vi "VariableGroupsEditUI.vi"(11 "VariableManagerRef in":refnum<vi>) -> (3 "VariableManagerRef out":refnum<vi>)   [LabVIEW 2013]
doc: "Create a window for add/edit variable groups of the given VariableManager reference."
uses:
  VariableGroup/VariableGroup.lvclass
  VariableManager/VariableManager.lvclass
  Variable/Variable.lvclass
  API/VariableManagerAPI.lvlib
panel:
  in  "Delete Button":bool
  in  "Rename Button":bool
  in  "Add Button":bool
  in  "InputName":string caption="Input Group Name"
  in  "VariableNames":string[](array[string])
  in  "VariableGroups":refnum<class "VariableGroup.lvclass">[](array[class])
  in  "OK Button":bool
  in  "Cancel Button":bool
  in  "Exclude":bool
  in  "Include":bool
  in  "IncludedVariables":i32[](listbox) caption="Included Variables"
  in  "ExcludedVariables":i32[](listbox) caption="Excluded Variables"
  in  "VariableGroup":u16(ring) caption="Variable Group"
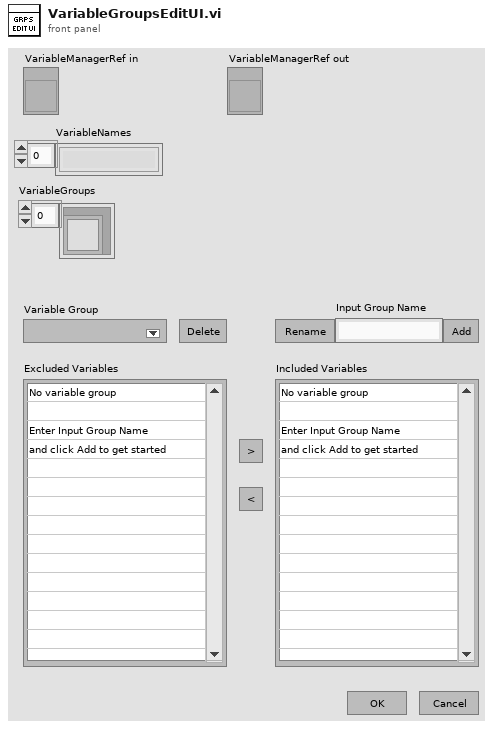
[diagram p1: front panel]
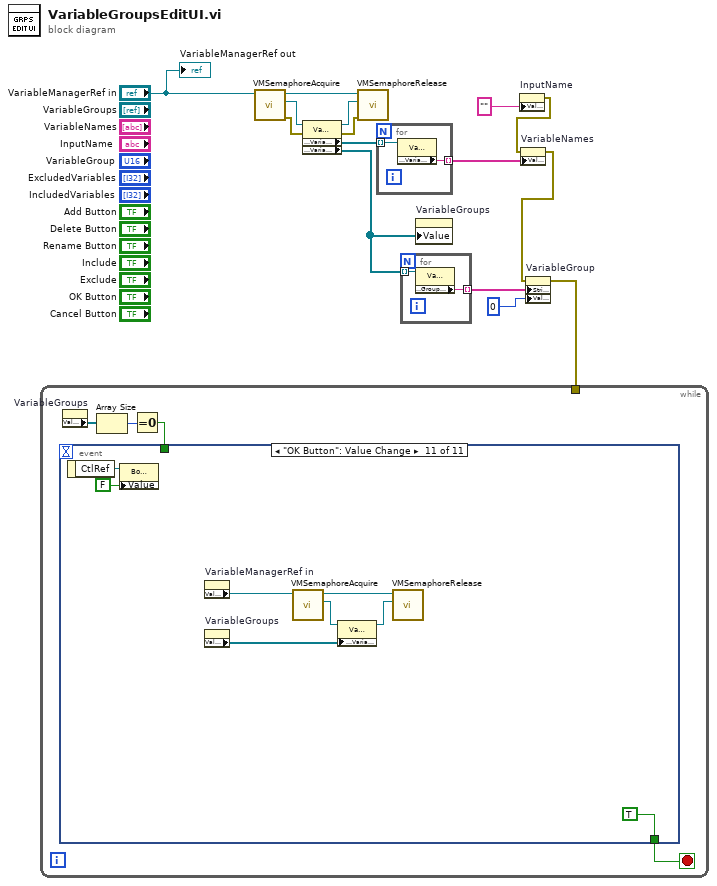
[diagram p0: block diagram]
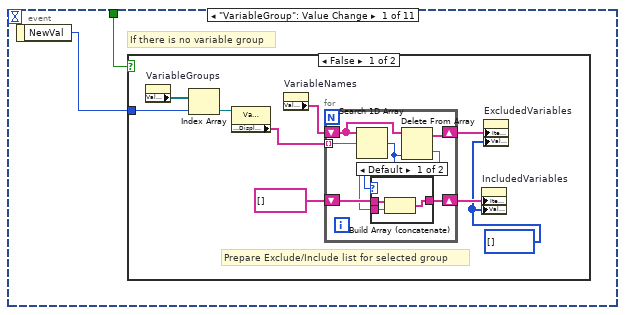
[diagram p2: hidden frame]
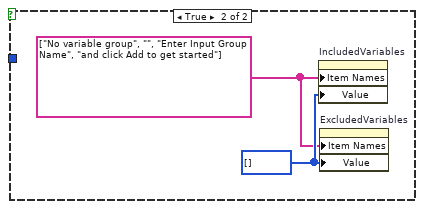
[diagram p4: hidden frame]
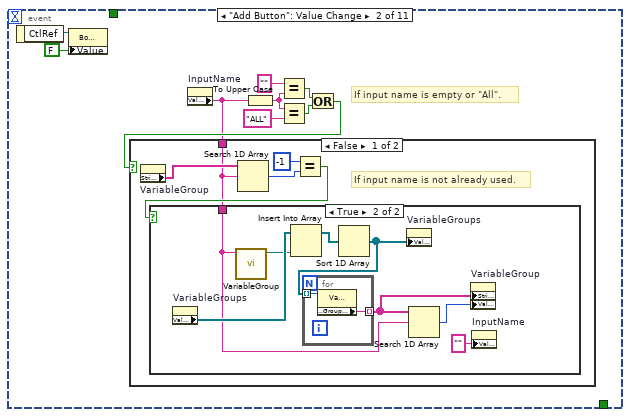
[diagram p5: hidden frame]
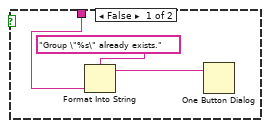
[diagram p6: hidden frame]
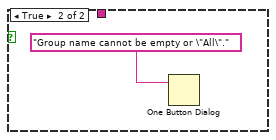
[diagram p7: hidden frame]
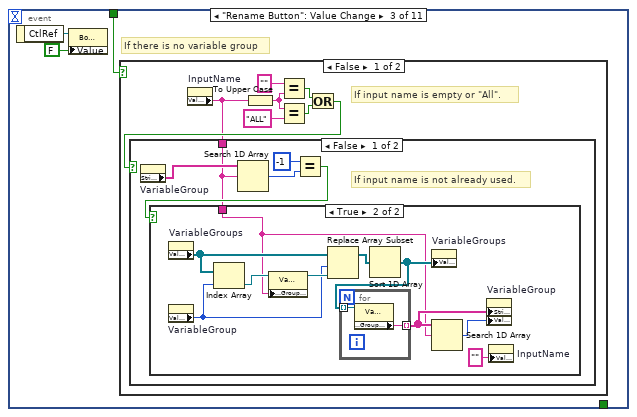
[diagram p8: hidden frame]
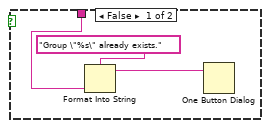
[diagram p9: hidden frame]
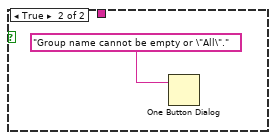
[diagram p10: hidden frame]
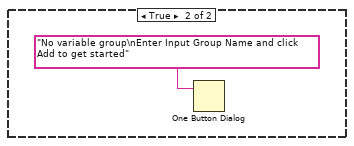
[diagram p11: hidden frame]
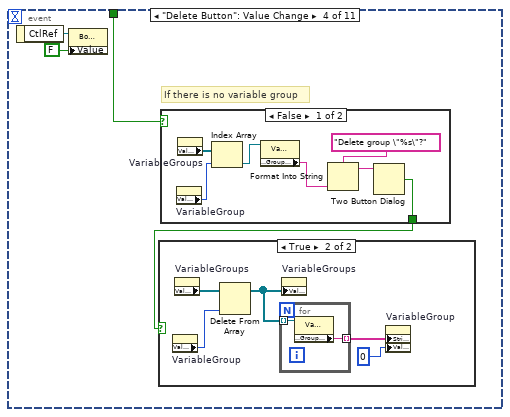
[diagram p12: hidden frame]
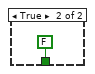
[diagram p13: hidden frame]
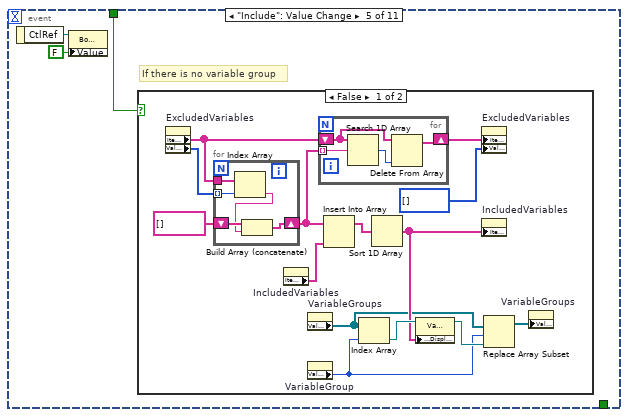
[diagram p15: hidden frame]
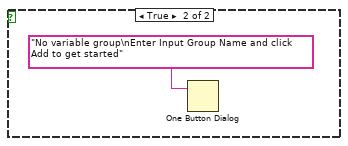
[diagram p16: hidden frame]
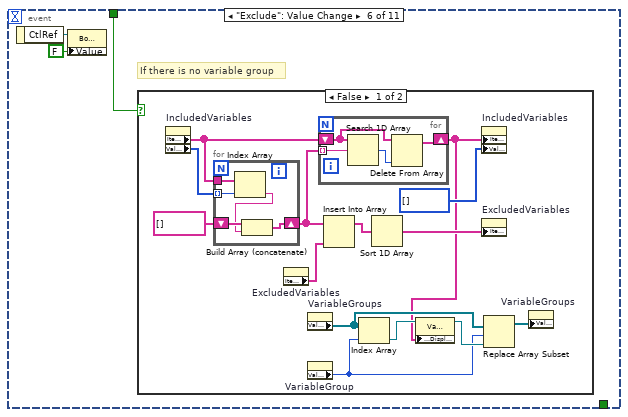
[diagram p17: hidden frame]
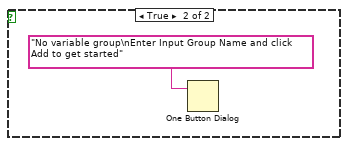
[diagram p18: hidden frame]
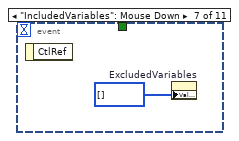
[diagram p19: hidden frame]
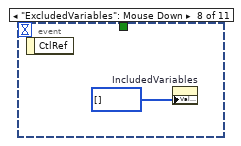
[diagram p20: hidden frame]
diagram:
  n1 = call "VMSemaphoreAcquire.vi"("VariableManagerRef in"="VariableManagerRef in") -> ("error out"=w2:errorcluster, "VariableManager"=w10:refnum<class "VariableManager.lvclass">, "VariableManagerRef out"=w4:refnum<vi>)  [unwired: 7 in, 1 out]
  n2 = property class="VariableManager.lvclass"(reference=w10, error in=w2) -> (reference out=w5:refnum<class "VariableManager.lvclass">, error out=w1:errorcluster, "Accessors:Variables"=w8:refnum<class "Variable.lvclass">[], "Accessors:VariableGroups"=w9:refnum<class "VariableGroup.lvclass">[])
  n3 = call "VMSemaphoreRelease.vi"("error in (no error)"=w1, "VariableManager"=w5, "VariableManagerRef in"=w4) -> ()  [unwired: 7 in, 2 out]
  n4 = for {
    tunnel: w8 -> [w17] mode=indexing
    tunnel: [w16] -> w7 mode=indexing
    n5 = property class="Variable.lvclass"(reference=w17) -> ("Accessors:VariableName"=w16:string)  [unwired: 1 in, 2 out]
  }
  n6 = for {
    tunnel: w9 -> [w19] mode=indexing
    tunnel: [w18] -> w14 mode=indexing
    n7 = property class="VariableGroup.lvclass"(reference=w19) -> ("Accessors:GroupName"=w18:string)  [unwired: 1 in, 2 out]
  }
  n8 = property on="VariableGroups" class="Arr (strict)"("Value"=w9) -> ()  [unwired: 2 in, 2 out]
  n9 = property on="InputName" class="Str"("Value"="") -> (error out=w11:errorcluster)  [unwired: 2 in, 1 out]
  n10 = property on="VariableNames" class="Arr (strict)"(error in=w11, "Value"=w7) -> (error out=w13:errorcluster)  [unwired: 1 in, 1 out]
  n11 = property on="VariableGroup" class="Ring (strict)"(error in=w13, "Strings []"=w14, "Val(Sgnl)"=u16 0 ("Value (Signaling)")) -> (error out=w6:errorcluster)  [unwired: 1 in, 1 out]
  n12 = while {
    tunnel: w6 -> [_]
    stop <- w23 stop-if-true
    n13 = property on="VariableGroups" class="Arr (strict)"() -> ("Value"=w21:refnum<class "VariableGroup.lvclass">[])  [unwired: 2 in, 2 out]
    n14 = Array Size(array=w21) -> (size(s)=w22:i32)
    n15 = Equal To 0?(x=w22) -> (x = 0?=w20:bool)
    n16 = event shown="[10] \"OK Button\": Value Change" {
      selector: _ -> [_ _ _ _ _ _ _ _ _ _ _]
      dyn-events: _ -> [_ _ _ _ _ _ _ _ _ _ _]
      timeout: _ -> [_ _ _ _ _ _ _ _ _ _ _]
      tunnel: [_ _ _ _ _ _ _ _ w186 w189 TRUE] -> w23
      tunnel: w20 -> [w24 _ w76 w108 w127 w154 _ _ _ _ _]
      event "VariableGroup": Value Change {
        # "If there is no variable group"
        n17 = event-data() -> ("NewVal"=w25:u16)  [unwired: 1 in]
        n18 = case shown="False" w24 {
          tunnel: w25 -> [w34 _]
          frame False {
            w26 = i32[] [] ("Exclude Variables")
            # "Prepare Exclude/Include list for selected group"
            n19 = property on="VariableGroups" class="Arr (strict)"() -> ("Value"=w29:refnum<class "VariableGroup.lvclass">[])  [unwired: 2 in, 2 out]
            n20 = Index Array(array=w29, index=w34) -> (element=w33:refnum<class "VariableGroup.lvclass">)
            n21 = property class="VariableGroup.lvclass"(reference=w33) -> ("Accessors:DisplayList"=w32:string[])  [unwired: 1 in, 2 out]
            n22 = property on="VariableNames" class="Arr (strict)"() -> ("Value"=w31:string[])  [unwired: 2 in, 2 out]
            n23 = for {
              tunnel: w32 -> [w41] mode=indexing
              shift-right: [w39] -> w30
              shift-left: w31 -> [w40]
              shift-right: [w38] -> w27
              shift-left: string[] [] -> [w37]
              n24 = Search 1D Array(1D array=w40, element=w41) -> (index of element=w36:i32)  [unwired: 1 in]
              n25 = Delete From Array(array=w40, index=w36) -> (deleted portion=w35:string, array with subset deleted=w39:string[])  [unwired: 1 in]
              n26 = case shown="Default" w36 {
                tunnel: [w44 w45] -> w38
                tunnel: w37 -> [w43 w45]
                tunnel: w35 -> [w42 _]
                frame Default {
                  n27 = Build Array (concatenate)(w43, w42) -> (w44:string[])
                }
                frame -1 {
                }
              }
            }
            n28 = property on="IncludedVariables" class="LstBox (strict)"("Item Names"=w27, "Value"=w26) -> ()  [unwired: 2 in, 2 out]
            n29 = property on="ExcludedVariables" class="LstBox (strict)"("Item Names"=w30, "Value"=w26) -> ()  [unwired: 2 in, 2 out]
          }
          frame True {
            w46 = string[] ["No variable group", "", "Enter Input Group Name", "and click Add to get started"] ("Item Names")
            w47 = i32[] [] ("Include Variables")
            n30 = property on="IncludedVariables" class="LstBox (strict)"("Item Names"=w46, "Value"=w47) -> ()  [unwired: 2 in, 2 out]
            n31 = property on="ExcludedVariables" class="LstBox (strict)"("Item Names"=w46, "Value"=w47) -> ()  [unwired: 2 in, 2 out]
          }
        }
      }
      event "Add Button": Value Change {
        # "If input name is empty or \"All\"."
        n32 = event-data() -> ("CtlRef"=w53:refnum<vi>)  [unwired: 1 in]
        n33 = property class="Bool (strict)"(reference=w53, "Value"=FALSE) -> ()  [unwired: 1 in, 2 out]
        n34 = property on="InputName" class="Str"() -> ("Value"=w52:string)  [unwired: 2 in, 2 out]
        n35 = To Upper Case(1:w52) -> (0:w48:string)
        n36 = Equal?(x="", y=w48) -> (x = y?=w49:bool)
        n37 = Equal?(x=w48, y="ALL") -> (x = y?=w50:bool)
        n38 = Or(x=w49, y=w50) -> (x .or. y?=w54:bool)
        n39 = case shown="False" w54 {
          tunnel: w52 -> [w59 _]
          frame False {
            # "If input name is not already used."
            n40 = property on="VariableGroup" class="Ring (strict)"() -> ("Strings []"=w61:string[])  [unwired: 2 in, 2 out]
            n41 = Search 1D Array(1D array=w61, element=w59) -> (index of element=w57:i32)  [unwired: 1 in]
            n42 = Equal?(x=-1 ("y"), y=w57) -> (x = y?=w60:bool)
            n43 = case shown="True" w60 {
              tunnel: w59 -> [w62 w67]
              frame False {
                n44 = Format Into String(format string="Group \"%s\" already exists.", w62) -> (resulting string=w63:string)  [unwired: 2 in, 1 out]
                n45 = One Button Dialog(message=w63) -> ()  [unwired: 1 in, 1 out]
              }
              frame True {
                n46 = property on="VariableGroups" class="Arr (strict)"() -> ("Value"=w72:refnum<class "VariableGroup.lvclass">[])  [unwired: 2 in, 2 out]
                n47 = call "VariableGroup.vi"("GroupName"=w67) -> ("VariableGroup"=w66:refnum<class "VariableGroup.lvclass">)  [unwired: 10 in]
                n48 = Insert Into Array(array=w72, new element=w66) -> (w71:refnum<class "VariableGroup.lvclass">[])  [unwired: 1 in]
                n49 = Sort 1D Array(array=w71) -> (sorted array=w70:refnum<class "VariableGroup.lvclass">[])
                n50 = for {
                  tunnel: w70 -> [w74] mode=indexing
                  tunnel: [w73] -> w69 mode=indexing
                  n51 = property class="VariableGroup.lvclass"(reference=w74) -> ("Accessors:GroupName"=w73:string)  [unwired: 1 in, 2 out]
                }
                n52 = property on="VariableGroups" class="Arr (strict)"("Value"=w70) -> ()  [unwired: 2 in, 2 out]
                n53 = Search 1D Array(1D array=w69, element=w67) -> (index of element=w68:i32)  [unwired: 1 in]
                n54 = property on="VariableGroup" class="Ring (strict)"("Strings []"=w69, "Val(Sgnl)"=w68) -> ()  [unwired: 2 in, 2 out]
                n55 = property on="InputName" class="Str"("Value"="") -> ()  [unwired: 2 in, 2 out]
              }
            }
          }
          frame True {
            n56 = One Button Dialog(message="Group name cannot be empty or \"All\".") -> ()  [unwired: 1 in, 1 out]
          }
        }
      }
      event "Rename Button": Value Change {
        # "If there is no variable group"
        n57 = event-data() -> ("CtlRef"=w78:refnum<vi>)  [unwired: 1 in]
        n58 = property class="Bool (strict)"(reference=w78, "Value"=FALSE) -> ()  [unwired: 1 in, 2 out]
        n59 = case shown="False" w76 {
          frame False {
            # "If input name is empty or \"All\"."
            n60 = property on="InputName" class="Str"() -> ("Value"=w83:string)  [unwired: 2 in, 2 out]
            n61 = To Upper Case(1:w83) -> (0:w79:string)
            n62 = Equal?(x="", y=w79) -> (x = y?=w80:bool)
            n63 = Equal?(x=w79, y="ALL") -> (x = y?=w81:bool)
            n64 = Or(x=w80, y=w81) -> (x .or. y?=w84:bool)
            n65 = case shown="False" w84 {
              tunnel: w83 -> [w88 _]
              frame False {
                # "If input name is not already used."
                n66 = property on="VariableGroup" class="Ring (strict)"() -> ("Strings []"=w90:string[])  [unwired: 2 in, 2 out]
                n67 = Search 1D Array(1D array=w90, element=w88) -> (index of element=w86:i32)  [unwired: 1 in]
                n68 = Equal?(x=-1 ("y"), y=w86) -> (x = y?=w89:bool)
                n69 = case shown="True" w89 {
                  tunnel: w88 -> [w91 w94]
                  frame False {
                    n70 = Format Into String(format string="Group \"%s\" already exists.", w91) -> (resulting string=w92:string)  [unwired: 2 in, 1 out]
                    n71 = One Button Dialog(message=w92) -> ()  [unwired: 1 in, 1 out]
                  }
                  frame True {
                    n72 = property on="VariableGroups" class="Arr (strict)"() -> ("Value"=w100:refnum<class "VariableGroup.lvclass">[])  [unwired: 2 in, 2 out]
                    n73 = property on="VariableGroup" class="Ring (strict)"() -> ("Value"=w98:u16)  [unwired: 2 in, 2 out]
                    n74 = Index Array(array=w100, index=w98) -> (element=w101:refnum<class "VariableGroup.lvclass">)
                    n75 = property class="VariableGroup.lvclass"(reference=w101, "Accessors:GroupName"=w94) -> (reference out=w99:refnum<class "VariableGroup.lvclass">)  [unwired: 1 in, 1 out]
                    n76 = Replace Array Subset(array=w100, new element=w99, index=w98) -> (w97:refnum<class "VariableGroup.lvclass">[])
                    n77 = Sort 1D Array(array=w97) -> (sorted array=w96:refnum<class "VariableGroup.lvclass">[])
                    n78 = for {
                      tunnel: w96 -> [w105] mode=indexing
                      tunnel: [w104] -> w103 mode=indexing
                      n79 = property class="VariableGroup.lvclass"(reference=w105) -> ("Accessors:GroupName"=w104:string)  [unwired: 1 in, 2 out]
                    }
                    n80 = property on="VariableGroups" class="Arr (strict)"("Value"=w96) -> ()  [unwired: 2 in, 2 out]
                    n81 = Search 1D Array(1D array=w103, element=w94) -> (index of element=w102:i32)  [unwired: 1 in]
                    n82 = property on="VariableGroup" class="Ring (strict)"("Strings []"=w103, "Val(Sgnl)"=w102) -> ()  [unwired: 2 in, 2 out]
                    n83 = property on="InputName" class="Str"("Value"="") -> ()  [unwired: 2 in, 2 out]
                  }
                }
              }
              frame True {
                n84 = One Button Dialog(message="Group name cannot be empty or \"All\".") -> ()  [unwired: 1 in, 1 out]
              }
            }
          }
          frame True {
            n85 = One Button Dialog(message="No variable group\nEnter Input Group Name and click Add to get started") -> ()  [unwired: 1 in, 1 out]
          }
        }
      }
      event "Delete Button": Value Change {
        # "If there is no variable group"
        n86 = event-data() -> ("CtlRef"=w111:refnum<vi>)  [unwired: 1 in]
        n87 = property class="Bool (strict)"(reference=w111, "Value"=FALSE) -> ()  [unwired: 1 in, 2 out]
        n88 = case shown="False" w108 {
          tunnel: [w112 FALSE ("T button?")] -> w109
          frame False {
            n89 = property on="VariableGroup" class="Ring (strict)"() -> ("Value"=w118:u16)  [unwired: 2 in, 2 out]
            n90 = property on="VariableGroups" class="Arr (strict)"() -> ("Value"=w117:refnum<class "VariableGroup.lvclass">[])  [unwired: 2 in, 2 out]
            n91 = Index Array(array=w117, index=w118) -> (element=w116:refnum<class "VariableGroup.lvclass">)
            n92 = property class="VariableGroup.lvclass"(reference=w116) -> ("Accessors:GroupName"=w114:string)  [unwired: 1 in, 2 out]
            n93 = Format Into String(format string="Delete group \"%s\"?", w114) -> (resulting string=w113:string)  [unwired: 2 in, 1 out]
            n94 = Two Button Dialog(message=w113) -> (T button?=w112:bool)  [unwired: 2 in]
          }
          frame True {
          }
        }
        n95 = case shown="True" w109 {
          frame False {
          }
          frame True {
            n96 = property on="VariableGroup" class="Ring (strict)"() -> ("Value"=w122:u16)  [unwired: 2 in, 2 out]
            n97 = property on="VariableGroups" class="Arr (strict)"() -> ("Value"=w124:refnum<class "VariableGroup.lvclass">[])  [unwired: 2 in, 2 out]
            n98 = Delete From Array(array=w124, index=w122) -> (array with subset deleted=w121:refnum<class "VariableGroup.lvclass">[])  [unwired: 1 in, 1 out]
            n99 = for {
              tunnel: w121 -> [w126] mode=indexing
              tunnel: [w125] -> w123 mode=indexing
              n100 = property class="VariableGroup.lvclass"(reference=w126) -> ("Accessors:GroupName"=w125:string)  [unwired: 1 in, 2 out]
            }
            n101 = property on="VariableGroups" class="Arr (strict)"("Value"=w121) -> ()  [unwired: 2 in, 2 out]
            n102 = property on="VariableGroup" class="Ring (strict)"("Strings []"=w123, "Val(Sgnl)"=u16 0 ("Value (Signaling)")) -> ()  [unwired: 2 in, 2 out]
          }
        }
      }
      event "Include": Value Change {
        # "If there is no variable group"
        n103 = event-data() -> ("CtlRef"=w129:refnum<vi>)  [unwired: 1 in]
        n104 = property class="Bool (strict)"(reference=w129, "Value"=FALSE) -> ()  [unwired: 1 in, 2 out]
        n105 = case shown="False" w127 {
          frame False {
            n106 = property on="ExcludedVariables" class="LstBox (strict)"() -> ("Item Names"=w133:string[], "Value"=w142:i32[])  [unwired: 2 in, 2 out]
            n107 = for {
              tunnel: w142 -> [w149] mode=indexing
              shift-right: [w151] -> w132
              shift-left: string[] [] -> [w152]
              tunnel: w133 -> [w150]
              n108 = Index Array(array=w150, index=w149) -> (element=w148:string)
              n109 = Build Array (concatenate)(w152, w148) -> (w151:string[])
            }
            n110 = property on="IncludedVariables" class="LstBox (strict)"() -> ("Item Names"=w140:string[])  [unwired: 2 in, 2 out]
            n111 = property on="VariableGroups" class="Arr (strict)"() -> ("Value"=w137:refnum<class "VariableGroup.lvclass">[])  [unwired: 2 in, 2 out]
            n112 = property on="VariableGroup" class="Ring (strict)"() -> ("Value"=w135:u16)  [unwired: 2 in, 2 out]
            n113 = for {
              tunnel: w132 -> [w147] mode=indexing
              shift-right: [w144] -> w131
              shift-left: w133 -> [w145]
              n114 = Search 1D Array(1D array=w145, element=w147) -> (index of element=w146:i32)  [unwired: 1 in]
              n115 = Delete From Array(array=w145, index=w146) -> (array with subset deleted=w144:string[])  [unwired: 1 in, 1 out]
            }
            n116 = Insert Into Array(array=w132, new element=w140) -> (w139:string[])  [unwired: 1 in]
            n117 = Index Array(array=w137, index=w135) -> (element=w143:refnum<class "VariableGroup.lvclass">)
            n118 = Sort 1D Array(array=w139) -> (sorted array=w138:string[])
            n119 = property class="VariableGroup.lvclass"(reference=w143, "Accessors:DisplayList"=w138) -> (reference out=w136:refnum<class "VariableGroup.lvclass">)  [unwired: 1 in, 1 out]
            n120 = property on="ExcludedVariables" class="LstBox (strict)"("Item Names"=w131, "Value"=i32[] [] ("Exclude Variables")) -> ()  [unwired: 2 in, 2 out]
            n121 = property on="IncludedVariables" class="LstBox (strict)"("Item Names"=w138) -> ()  [unwired: 2 in, 2 out]
            n122 = Replace Array Subset(array=w137, new element=w136, index=w135) -> (w134:refnum<class "VariableGroup.lvclass">[])
            n123 = property on="VariableGroups" class="Arr (strict)"("Value"=w134) -> ()  [unwired: 2 in, 2 out]
          }
          frame True {
            n124 = One Button Dialog(message="No variable group\nEnter Input Group Name and click Add to get started") -> ()  [unwired: 1 in, 1 out]
          }
        }
      }
      event "Exclude": Value Change {
        # "If there is no variable group"
        n125 = event-data() -> ("CtlRef"=w156:refnum<vi>)  [unwired: 1 in]
        n126 = property class="Bool (strict)"(reference=w156, "Value"=FALSE) -> ()  [unwired: 1 in, 2 out]
        n127 = case shown="False" w154 {
          frame False {
            n128 = property on="IncludedVariables" class="LstBox (strict)"() -> ("Item Names"=w161:string[], "Value"=w160:i32[])  [unwired: 2 in, 2 out]
            n129 = for {
              tunnel: w160 -> [w176] mode=indexing
              shift-right: [w178] -> w163
              shift-left: string[] [] -> [w179]
              tunnel: w161 -> [w177]
              n130 = Index Array(array=w177, index=w176) -> (element=w175:string)
              n131 = Build Array (concatenate)(w179, w175) -> (w178:string[])
            }
            n132 = property on="ExcludedVariables" class="LstBox (strict)"() -> ("Item Names"=w162:string[])  [unwired: 2 in, 2 out]
            n133 = property on="VariableGroups" class="Arr (strict)"() -> ("Value"=w167:refnum<class "VariableGroup.lvclass">[])  [unwired: 2 in, 2 out]
            n134 = property on="VariableGroup" class="Ring (strict)"() -> ("Value"=w165:u16)  [unwired: 2 in, 2 out]
            n135 = for {
              tunnel: w163 -> [w174] mode=indexing
              shift-right: [w171] -> w157
              shift-left: w161 -> [w172]
              n136 = Search 1D Array(1D array=w172, element=w174) -> (index of element=w173:i32)  [unwired: 1 in]
              n137 = Delete From Array(array=w172, index=w173) -> (array with subset deleted=w171:string[])  [unwired: 1 in, 1 out]
            }
            n138 = Insert Into Array(array=w163, new element=w162) -> (w168:string[])  [unwired: 1 in]
            n139 = Index Array(array=w167, index=w165) -> (element=w170:refnum<class "VariableGroup.lvclass">)
            n140 = Sort 1D Array(array=w168) -> (sorted array=w158:string[])
            n141 = property class="VariableGroup.lvclass"(reference=w170, "Accessors:DisplayList"=w157) -> (reference out=w166:refnum<class "VariableGroup.lvclass">)  [unwired: 1 in, 1 out]
            n142 = property on="IncludedVariables" class="LstBox (strict)"("Item Names"=w157, "Value"=i32[] [] ("Exclude Variables")) -> ()  [unwired: 2 in, 2 out]
            n143 = property on="ExcludedVariables" class="LstBox (strict)"("Item Names"=w158) -> ()  [unwired: 2 in, 2 out]
            n144 = Replace Array Subset(array=w167, new element=w166, index=w165) -> (w164:refnum<class "VariableGroup.lvclass">[])
            n145 = property on="VariableGroups" class="Arr (strict)"("Value"=w164) -> ()  [unwired: 2 in, 2 out]
          }
          frame True {
            n146 = One Button Dialog(message="No variable group\nEnter Input Group Name and click Add to get started") -> ()  [unwired: 1 in, 1 out]
          }
        }
      }
      event "IncludedVariables": Mouse Down {
        n147 = event-data() -> ()  [unwired: 1 in, 1 out]
        n148 = property on="ExcludedVariables" class="LstBox (strict)"("Value"=i32[] [] ("Exclude Variables")) -> ()  [unwired: 2 in, 2 out]
      }
      event "ExcludedVariables": Mouse Down {
        n149 = event-data() -> ()  [unwired: 1 in, 1 out]
        n150 = property on="IncludedVariables" class="LstBox (strict)"("Value"=i32[] [] ("Exclude Variables")) -> ()  [unwired: 2 in, 2 out]
      }
      event "Cancel Button": Value Change {
        n151 = event-data() -> ("CtlRef"=w188:refnum<vi>)  [unwired: 1 in]
        n152 = property class="Bool (strict)"(reference=w188, "Value"=FALSE) -> ()  [unwired: 1 in, 2 out]
        n153 = Two Button Dialog(message="Discard all changes and close this window?", 1:"No", 2:"Yes") -> (T button?=w186:bool)
      }
      event Panel Close? {
        n154 = event-data() -> ()  [unwired: 1 in, 1 out]
        n155 = Two Button Dialog(message="Discard all changes and close this window?", 1:"No", 2:"Yes") -> (T button?=w189:bool)
        n156 = Not(x=w189) -> (.not. x?=w190:bool)
        n157 = event-data("Discard?"=w190) -> ()  [unwired: 1 in, 1 out]
      }
      event "OK Button": Value Change {
        n158 = event-data() -> ("CtlRef"=w201:refnum<vi>)  [unwired: 1 in]
        n159 = property class="Bool (strict)"(reference=w201, "Value"=FALSE) -> ()  [unwired: 1 in, 2 out]
        n160 = property on="VariableManagerRef in" class="LVObjRef (strict)"() -> ("Value"=w194:refnum<vi>)  [unwired: 2 in, 2 out]
        n161 = property on="VariableGroups" class="Arr (strict)"() -> ("Value"=w195:refnum<class "VariableGroup.lvclass">[])  [unwired: 2 in, 2 out]
        n162 = call "VMSemaphoreAcquire.vi"("VariableManagerRef in"=w194) -> ("VariableManager"=w197:refnum<class "VariableManager.lvclass">, "VariableManagerRef out"=w198:refnum<vi>)  [unwired: 7 in, 2 out]
        n163 = property class="VariableManager.lvclass"(reference=w197, "Accessors:VariableGroups"=w195) -> (reference out=w196:refnum<class "VariableManager.lvclass">)  [unwired: 1 in, 1 out]
        n164 = call "VMSemaphoreRelease.vi"("VariableManager"=w196, "VariableManagerRef in"=w198) -> ()  [unwired: 8 in, 2 out]
      }
    }
  }
  "VariableManagerRef out" <- "VariableManagerRef in"
